vi "Build Control Word.vi"(8 "error in (no error)":errorcluster, 11 "Async Message in":refnum<class "Async Message.lvclass">) -> (0 "error out":errorcluster, 2 "Control Word":u16)   [LabVIEW 2020, in "BCI-1553 API.lvlib" / "Async Message.lvclass"]
doc: "Builds the asynchronous control word. This word needs to be returned to the caller. The outside world is responsible for writing this data out to the Holt IC."
uses:
  Async Message.lvclass
  Async Message.lvclass/Async Message.ctl
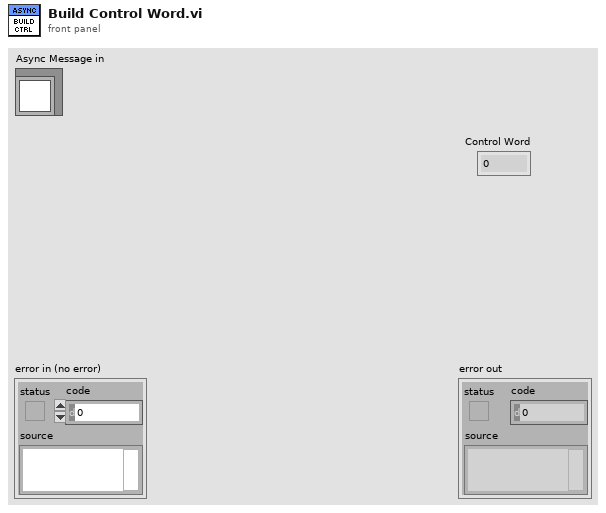
[diagram p1: front panel]
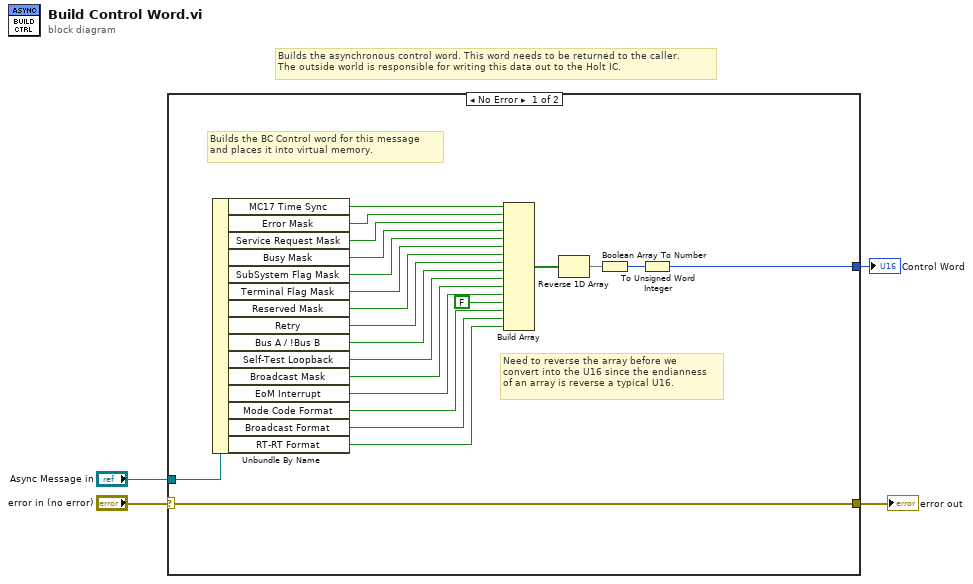
[diagram p0: block diagram]
diagram:
  # "Builds the asynchronous control word. This word needs to be returned to the caller.\nThe outside world is responsible for writing this data out to the Holt IC."
  n1 = case shown="No Error" "error in (no error)" {
    selector: "error in (no error)" -> [w26 w27]
    tunnel: [w26 w27] -> w2
    tunnel: "Async Message in" -> [w25 _]
    tunnel: [w5 _] -> w1
    frame No Error {
      # "Need to reverse the array before we\nconvert into the U16 since the endianness\nof an array is reverse a typical U16."
      # "Builds the BC Control word for this message\nand places it into virtual memory."
      n2 = Unbundle By Name(w25) -> ("MC17 Time Sync"=w6:bool, "Error Mask"=w12:bool, "Service Request Mask"=w13:bool, "Busy Mask"=w14:bool, "SubSystem Flag Mask"=w15:bool, "Terminal Flag Mask"=w16:bool, "Reserved Mask"=w17:bool, "Retry"=w18:bool, "Bus A / !Bus B"=w19:bool, "Self-Test Loopback"=w20:bool, "Broadcast Mask"=w21:bool, "EoM Interrupt"=w10:bool, "Mode Code Format"=w11:bool, "Broadcast Format"=w24:bool, "RT-RT Format"=w23:bool)
      n3 = Build Array(w6, w12, w13, w14, w15, w16, w17, w18, w19, w20, w21, w10, FALSE ("element"), w11, w24, w23) -> (w9:bool[])
      n4 = Reverse 1D Array(array=w9) -> (reversed array=w8:bool[])
      n5 = Boolean Array To Number(Boolean array=w8) -> (number=w7:u32)
      n6 = To Unsigned Word Integer(number=w7) -> (unsigned 16bit integer=w5:u16)
    }
    frame Error {
    }
  }
  "error out" <- w2
  "Control Word" <- w1
